vi "MATLAB_SCRIPT_CONCAT_STRING.vi"(0 "FILENAME":string, 1 "COLOR_STR":string, 4 "Line Style":string(combo)="-", 6 "Marker Shape":string(combo)="*", 7 "Wait":i32=3 min=0 max=15 step=1, 8 "Polydegree Line Width":i32=2 min=0 max=15 step=1, 9 "PolyDegree":i32=3 min=0 max=69 step=1, 10 "Line Width":i32=1 min=0 max=15 step=1, 11 "Marker Size":i32=2 min=1 max=15 step=1) -> (2 "SCRIPT_STR":string[](array[string]))   [LabVIEW 2013]
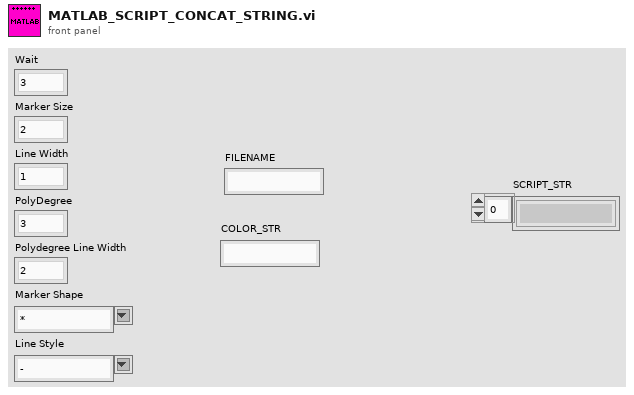
[diagram p1: front panel]
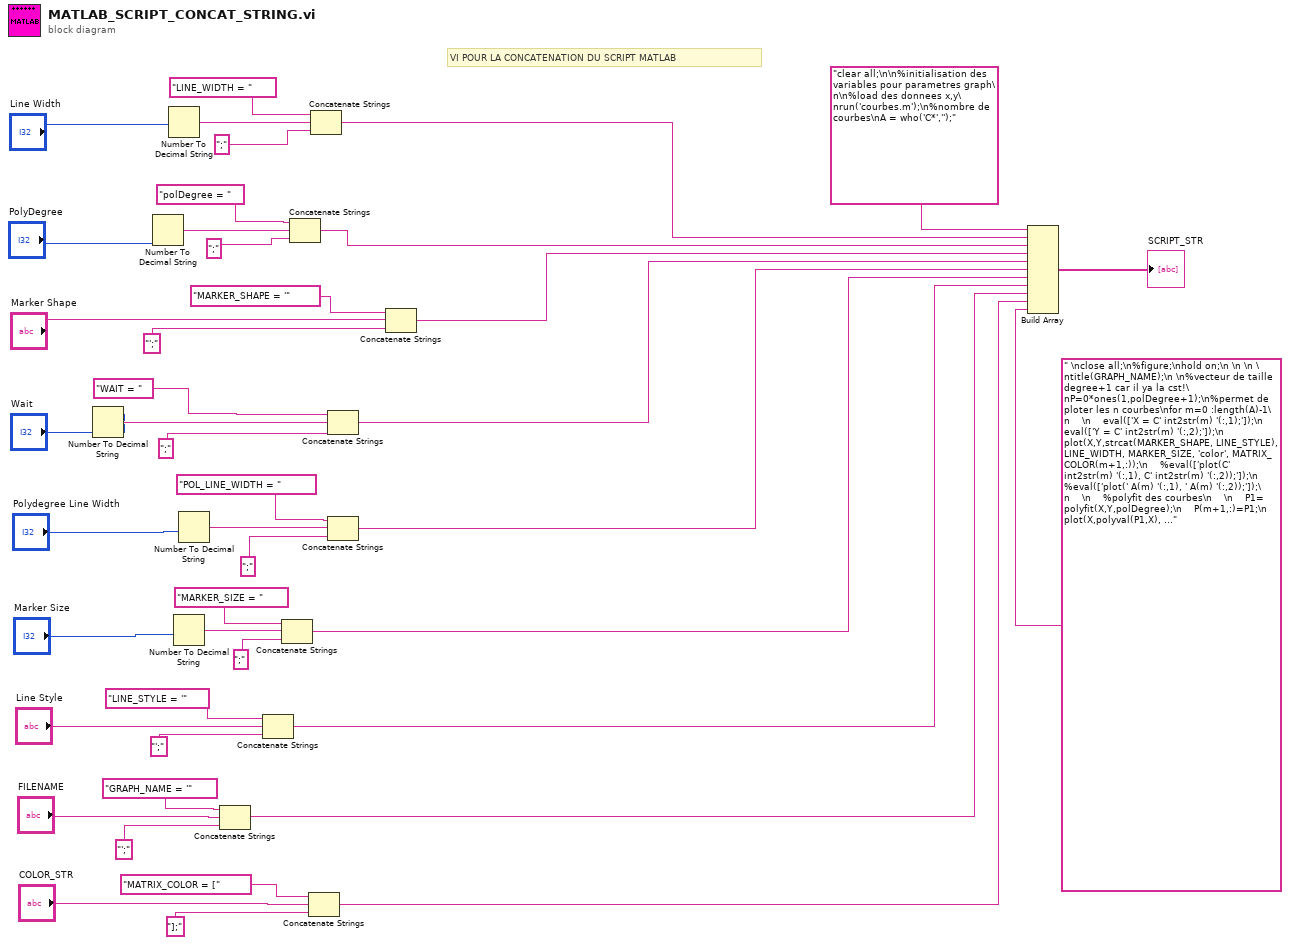
[diagram p0: block diagram]
diagram:
  # "VI POUR LA CONCATENATION DU SCRIPT MATLAB"
  n1 = Number To Decimal String(number="Wait") -> (decimal integer string=w34:string)  [unwired: 1 in]
  n2 = Number To Decimal String(number="PolyDegree") -> (decimal integer string=w38:string)  [unwired: 1 in]
  n3 = Number To Decimal String(number="Line Width") -> (decimal integer string=w41:string)  [unwired: 1 in]
  n4 = Number To Decimal String(number="Marker Size") -> (decimal integer string=w26:string)  [unwired: 1 in]
  n5 = Number To Decimal String(number="Polydegree Line Width") -> (decimal integer string=w30:string)  [unwired: 1 in]
  n6 = Concatenate Strings("GRAPH_NAME = '", "FILENAME", "';") -> (w8:string)
  n7 = Concatenate Strings("LINE_STYLE = '", "Line Style", "';") -> (w11:string)
  n8 = Concatenate Strings("MARKER_SIZE = ", w26, ";") -> (w12:string)
  n9 = Concatenate Strings("polDegree = ", w38, ";") -> (w16:string)
  n10 = Concatenate Strings("MATRIX_COLOR = [" ("string"), "COLOR_STR", "];" ("string")) -> (w5:string)
  n11 = Concatenate Strings("LINE_WIDTH = ", w41, ";") -> (w17:string)
  n12 = Concatenate Strings("WAIT = ", w34, ";") -> (w14:string)
  n13 = Concatenate Strings("POL_LINE_WIDTH = ", w30, ";") -> (w13:string)
  n14 = Concatenate Strings("MARKER_SHAPE = '", "Marker Shape", "';") -> (w15:string)
  n15 = Build Array("clear all;\n\n%initialisation des variables pour parametres graph\n\n%load des donnees x,y\nrun('courbes.m');\n%nombre de courbes\nA = who('C*','');", w17, w16, w15, w14, w13, w12, w11, w8, w5, " \nclose all;\n%figure;\nhold on;\n \n \n \ntitle(GRAPH_NAME);\n \n%vecteur de taille degree+1 car il ya la cst!\nP=0*ones(1,polDegree+1);\n%permet de ploter les n courbes\nfor m=0 :length(A)-1\n    \n    eval(['X = C' int2str(m) '(:,1);']);\n    eval(['Y = C' int2str(m) '(:,2);']);\n    plot(X,Y,strcat(MARKER_SHAPE, LINE_STYLE), LINE_WIDTH, MARKER_SIZE, 'color', MATRIX_COLOR(m+1,:));\n    %eval(['plot(C' int2str(m) '(:,1), C' int2str(m) '(:,2));']);\n    %eval(['plot(' A(m) '(:,1), ' A(m) '(:,2));']);\n    \n    %polyfit des courbes\n    \n    P1= polyfit(X,Y,polDegree);\n    P(m+1,:)=P1;\n    plot(X,polyval(P1,X), strcat(MARKER_SHAPE, LINE_STYLE), POL_LINE_WIDTH, MARKER_SIZE, 'color', MATRIX_COLOR(m+1,:));\n    \nend;\n \npause(WAIT);\n \nprint('-dpdf', strcat(GRAPH_NAME,'.pdf'));\nxlswrite('P',P);\nhold off;\nclose all;\n") -> (→"SCRIPT_STR":string[])
